vi "SVA 4MV6 T025(mimo) CCE.vi"() -> ()   [LabVIEW 2020]
uses:
  <vilib>/addons/Fuzzy Logic/TypeDefs/FL Defuzzification.ctl
  <vilib>/addons/Fuzzy Logic/TypeDefs/FL Antecedent Connective.ctl
  <vilib>/addons/Fuzzy Logic/TypeDefs/FL Consequent Implication.ctl
  <vilib>/addons/Fuzzy Logic/TypeDefs/FL Modifier.ctl
  <vilib>/addons/Fuzzy Logic/Membership/FL Create Membership Function (Triangle).vi
  <vilib>/addons/Fuzzy Logic/Membership/FL Create Membership Function (Trapezoid).vi
  <vilib>/addons/Fuzzy Logic/FL Fuzzy Controller (MIMO).vi
  <vilib>/addons/Fuzzy Logic/NI_Fuzzy_Logic_API.lvlib
panel:
  out "output values":dbl[](array[numeric])
  out "distancia":dbl(slide) scale=0.0..100.0
  out "angulo":dbl(knob) scale=-25.0..25.0
  in  "Reset":bool
  out "Motor Izquierda":dbl(slide) scale=-100.0..100.0
  out "Motor Derecha":dbl(slide) scale=-100.0..100.0
  out "Plano de trabajo":picture
  in  "stop":bool
  # "Ceballos Conde Emanuel\n4MV6\nSistemas de visión artificial\n2022/1"
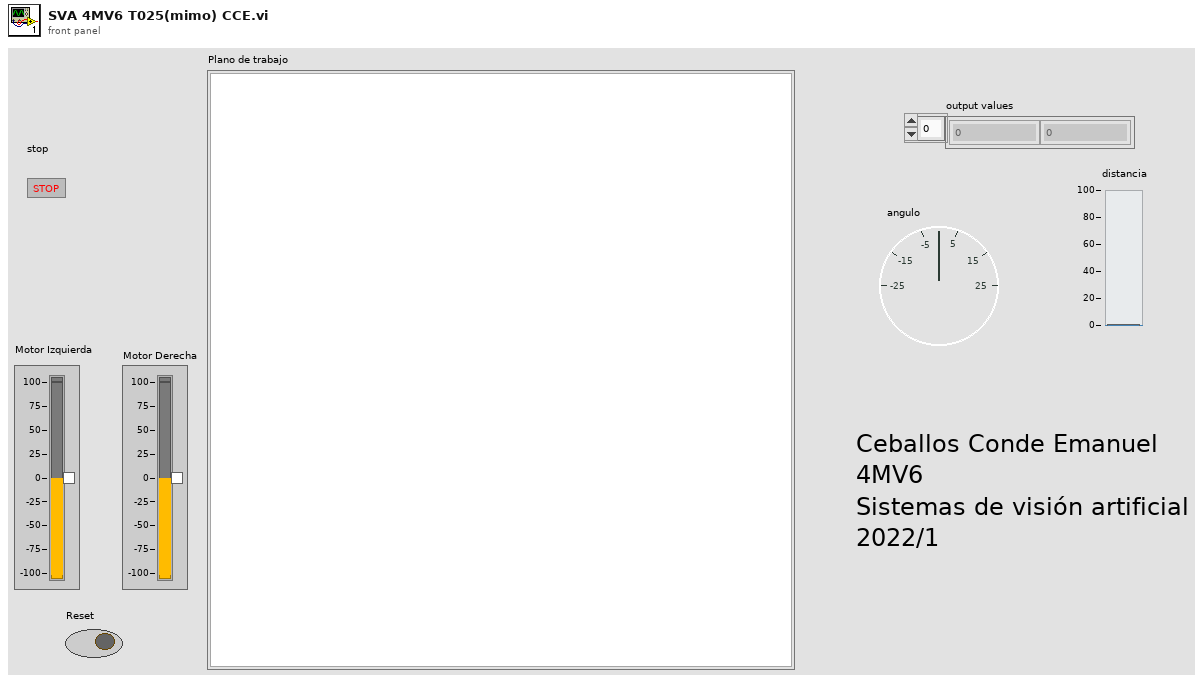
[diagram p1: front panel]
types:
  T1 = typedef "NI_Fuzzy_Logic_API.lvlib/FL Defuzzification.ctl" = u16
  T2 = typedef "NI_Fuzzy_Logic_API.lvlib/FL Membership Function.ctl" = cluster{"name":string, "shape":T3, "points":dbl[], "color":u32, "user-defined shape index":i32}
  T3 = typedef "NI_Fuzzy_Logic_API.lvlib/FL Membership Function Shape.ctl" = u16
  T4 = typedef "NI_Fuzzy_Logic_API.lvlib/FL Variable.ctl" = cluster{"name":string, "range":dbl[], "MFs":T2[]}
  T5 = typedef "NI_Fuzzy_Logic_API.lvlib/FL Modifier.ctl" = u16
  T6 = typedef "NI_Fuzzy_Logic_API.lvlib/FL Consequent Implication.ctl" = u16
  T7 = typedef "NI_Fuzzy_Logic_API.lvlib/FL Antecedent Connective.ctl" = u16
  T8 = typedef "NI_Fuzzy_Logic_API.lvlib/FL Consequent.ctl" = cluster{"Var Index":i32, "MF Index":i32, "Cond":T5}
  T9 = typedef "NI_Fuzzy_Logic_API.lvlib/FL Antecedent.ctl" = cluster{"Var Index":i32, "MF Index":i32, "Cond":T5}
  T10 = typedef "NI_Fuzzy_Logic_API.lvlib/FL Rule.ctl" = cluster{"antecedents":T9[], "antecedent connective":T7, "consequents":T8[], "consequent implication":T6, "degree of support":dbl}
  T11 = typedef "NI_Fuzzy_Logic_API.lvlib/FL System.ctl" = cluster{"input variables":T4[], "output variables":T4[], "rules":T10[], "defuzzification method":T1, "description":string, "user MF interpolating polynomials":T12[]}
  T12 = typedef "NI_Fuzzy_Logic_API.lvlib/FL Interpolating polynomials.ctl" = cluster{"X":dbl[], "Y":dbl[], "Y(x) coeff":dbl[][], "X(y) coeff":dbl[][], "Area(y) coeff":dbl[][], "coa_x(y) coeff":dbl[][]}
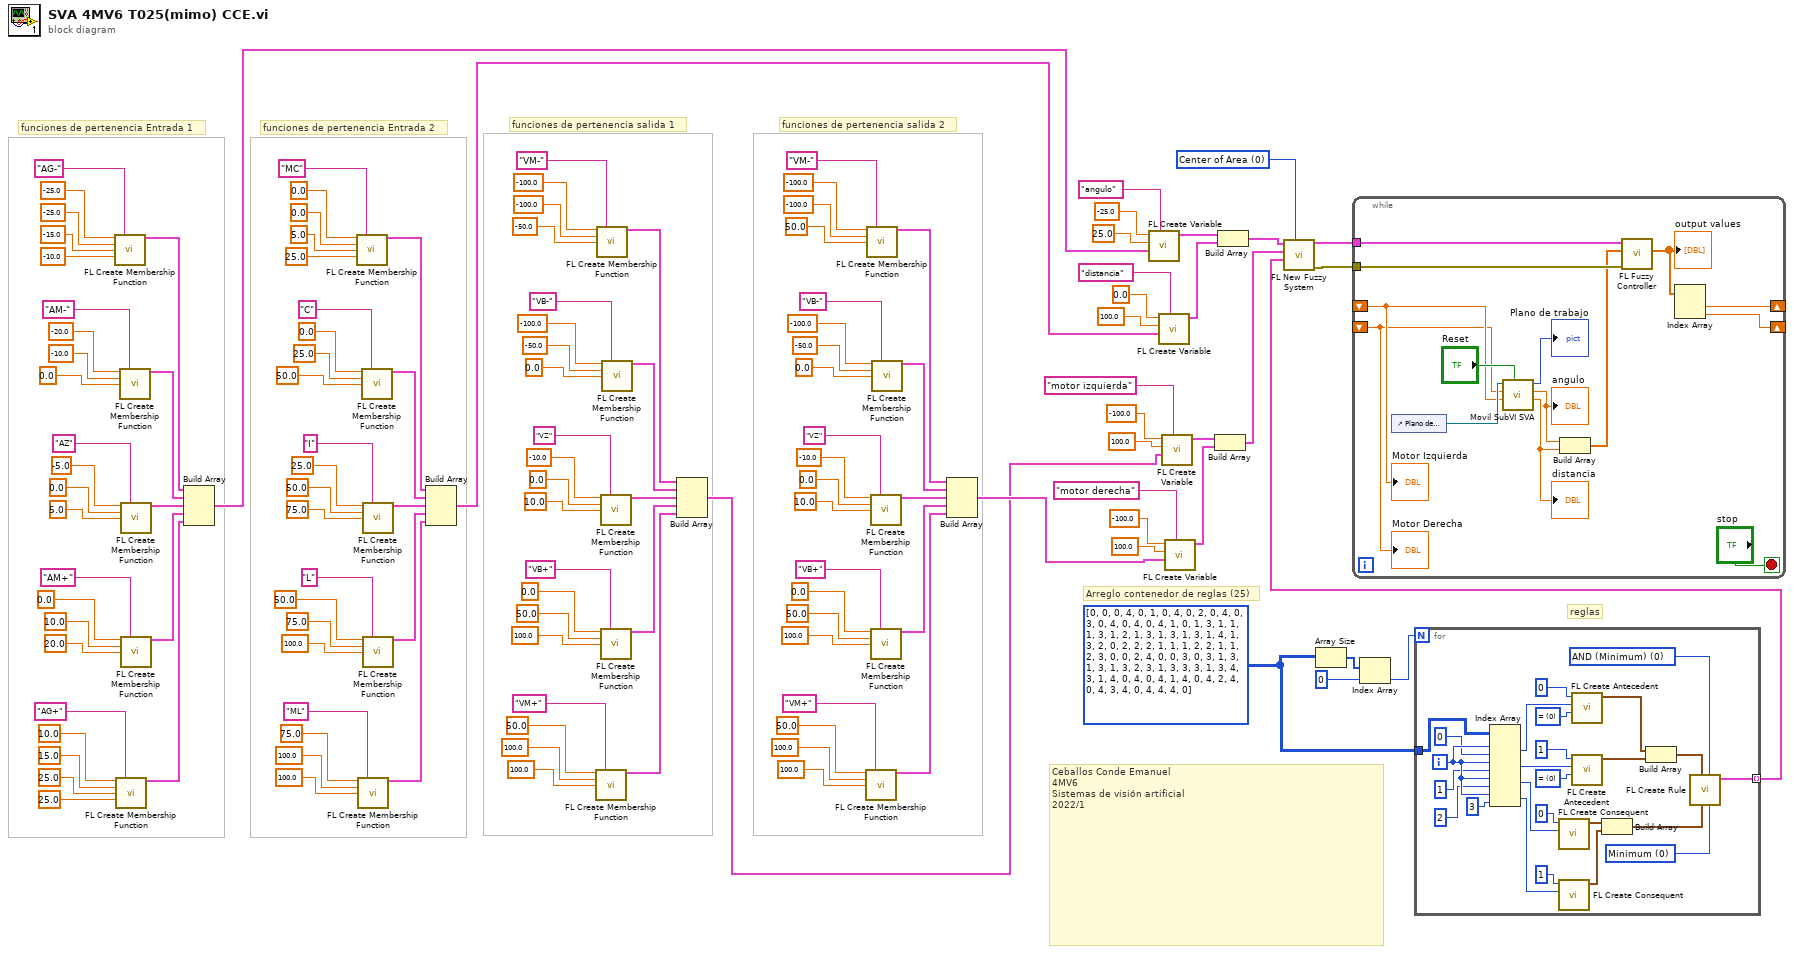
[diagram p0: block diagram]
diagram:
  w4 = i32[][] [[0, 0, 0, 4], [0, 1, 0, 4], [0, 2, 0, 4], [0, 3, 0, 4], [0, 4, 0, 4], [1, 0, 1, 3], [1, 1, 1, 3], [1, 2, 1, 3], [1, 3, 1, 3], [1, 4, 1, 3], [2, 0, 2, 2], [2, 1, 1, 1], [2, 2, 1, 1], [2, 3, 0, 0], [2, 4, 0, 0], [3, 0, 3, 1], [3, 1, 3, 1], [3, 2, 3, 1], [3, 3, 3, 1], [3, 4, 3, 1], [4, 0, 4, 0], [4, 1, 4, 0], [4, 2, 4, 0], [4, 3, 4, 0], [4, 4, 4, 0]]
  w131 = T1 0 items=["Center of Area", "Modified Center of Area", "Center of Sums", "Center of Maximum", "Mean of Maximum"] ("defuzzification method")
  # "Ceballos Conde Emanuel\n4MV6\nSistemas de visión artificial\n2022/1"
  # "Arreglo contenedor de reglas (25)"
  # "funciones de pertenencia salida 2"
  # "funciones de pertenencia salida 1"
  # "funciones de pertenencia Entrada 2"
  # "funciones de pertenencia Entrada 1"
  # "reglas"
  n1 = call-poly <vilib>:"FL Create Membership Function.vi"("left base"=-25.0, "name"="AG-", "left top"=-25.0 ("top"), "right top"=-15.0 ("right base"), "right base"=-10.0) -> ("membership function"=w107:T2)  [unwired: 9 in, 1 out]
  n2 = call-poly <vilib>:"FL Create Membership Function.vi"("left base"=10.0, "name"="AG+", "left top"=15.0 ("top"), "right top"=25.0 ("right base"), "right base"=25.0) -> ("membership function"=w87:T2)  [unwired: 9 in, 1 out]
  n3 = call-poly <vilib>:"FL Create Membership Function.vi"("left base"=-20.0, "name"="AM-", "top"=-10.0, "right base"=0.0) -> ("membership function"=w102:T2)  [unwired: 10 in, 1 out]
  n4 = call-poly <vilib>:"FL Create Membership Function.vi"("left base"=-5.0, "name"="AZ", "top"=0.0, "right base"=5.0) -> ("membership function"=w97:T2)  [unwired: 10 in, 1 out]
  n5 = call-poly <vilib>:"FL Create Membership Function.vi"("left base"=0.0, "name"="AM+", "top"=10.0, "right base"=20.0) -> ("membership function"=w92:T2)  [unwired: 10 in, 1 out]
  n6 = Build Array(w107, w102, w97, w92, w87) -> (w84:T2[])
  n7 = call-poly <vilib>:"FL Create Membership Function.vi"("left base"=0.0, "name"="MC", "left top"=0.0 ("top"), "right top"=5.0 ("right base"), "right base"=25.0) -> ("membership function"=w79:T2)  [unwired: 9 in, 1 out]
  n8 = call-poly <vilib>:"FL Create Membership Function.vi"("left base"=75.0, "name"="ML", "top"=100.0, "right base"=100.0) -> ("membership function"=w59:T2)  [unwired: 10 in, 1 out]
  n9 = call-poly <vilib>:"FL Create Membership Function.vi"("left base"=0.0, "name"="C", "top"=25.0, "right base"=50.0) -> ("membership function"=w74:T2)  [unwired: 10 in, 1 out]
  n10 = call-poly <vilib>:"FL Create Membership Function.vi"("left base"=25.0, "name"="I", "top"=50.0, "right base"=75.0) -> ("membership function"=w69:T2)  [unwired: 10 in, 1 out]
  n11 = call-poly <vilib>:"FL Create Membership Function.vi"("left base"=50.0, "name"="L", "top"=75.0, "right base"=100.0) -> ("membership function"=w64:T2)  [unwired: 10 in, 1 out]
  n12 = Build Array(w79, w74, w69, w64, w59) -> (w57:T2[])
  n13 = call-poly <vilib>:"FL Create Membership Function.vi"("left base"=50.0, "name"="VM+", "top"=100.0, "right base"=100.0) -> ("membership function"=w32:T2)  [unwired: 10 in, 1 out]
  n14 = call-poly <vilib>:"FL Create Membership Function.vi"("left base"=-100.0, "name"="VM-", "top"=-100.0, "right base"=-50.0) -> ("membership function"=w52:T2)  [unwired: 10 in, 1 out]
  n15 = call-poly <vilib>:"FL Create Membership Function.vi"("left base"=-10.0, "name"="VZ", "top"=0.0, "right base"=10.0) -> ("membership function"=w42:T2)  [unwired: 10 in, 1 out]
  n16 = call-poly <vilib>:"FL Create Membership Function.vi"("left base"=0.0, "name"="VB+", "top"=50.0, "right base"=100.0) -> ("membership function"=w37:T2)  [unwired: 10 in, 1 out]
  n17 = call-poly <vilib>:"FL Create Membership Function.vi"("left base"=-100.0, "name"="VB-", "top"=-50.0, "right base"=0.0) -> ("membership function"=w47:T2)  [unwired: 10 in, 1 out]
  n18 = Build Array(w52, w47, w42, w37, w32) -> (w5:T2[])
  n19 = call-poly <vilib>:"FL Create Membership Function.vi"("left base"=50.0, "name"="VM+", "top"=100.0, "right base"=100.0) -> ("membership function"=w7:T2)  [unwired: 10 in, 1 out]
  n20 = call-poly <vilib>:"FL Create Membership Function.vi"("left base"=-100.0, "name"="VM-", "top"=-100.0, "right base"=50.0) -> ("membership function"=w27:T2)  [unwired: 10 in, 1 out]
  n21 = call-poly <vilib>:"FL Create Membership Function.vi"("left base"=-10.0, "name"="VZ", "top"=0.0, "right base"=10.0) -> ("membership function"=w17:T2)  [unwired: 10 in, 1 out]
  n22 = call-poly <vilib>:"FL Create Membership Function.vi"("left base"=0.0, "name"="VB+", "top"=50.0, "right base"=100.0) -> ("membership function"=w12:T2)  [unwired: 10 in, 1 out]
  n23 = call-poly <vilib>:"FL Create Membership Function.vi"("left base"=-100.0, "name"="VB-", "top"=-50.0, "right base"=0.0) -> ("membership function"=w22:T2)  [unwired: 10 in, 1 out]
  n24 = Build Array(w27, w22, w17, w12, w7) -> (w6:T2[])
  n25 = call <vilib>:"FL Create Variable.vi"("name"="angulo", "membership functions"=w84, "maximum"=25.0, "minimum"=-25.0) -> ("variable"=w127:T4)  [unwired: 6 in, 1 out]
  n26 = call <vilib>:"FL Create Variable.vi"("name"="distancia", "membership functions"=w57, "maximum"=100.0, "minimum"=0.0) -> ("variable"=w114:T4)  [unwired: 6 in, 1 out]
  n27 = call <vilib>:"FL Create Variable.vi"("name"="motor izquierda", "membership functions"=w5, "maximum"=100.0, "minimum"=-100.0) -> ("variable"=w123:T4)  [unwired: 6 in, 1 out]
  n28 = call <vilib>:"FL Create Variable.vi"("name"="motor derecha", "membership functions"=w6, "maximum"=100.0, "minimum"=-100.0) -> ("variable"=w115:T4)  [unwired: 6 in, 1 out]
  n29 = Build Array(w123, w115) -> (w112:T4[])
  n30 = Build Array(w127, w114) -> (w113:T4[])
  n31 = Array Size(array=w4) -> (size(s)=w3:i32[])
  n32 = Index Array(array=w3, index=0) -> (element=w2:i32)
  n33 = for {
    N: w2 -> [_]
    tunnel: [w149] -> w119 mode=indexing
    tunnel: w4 -> [w134]
    i -> [w143]
    w147 = T5 0 items=["=", "!="] ("condition")
    w154 = T5 0 items=["=", "!="] ("condition")
    w157 = T6 0 items=["Minimum", "Product"] ("consequent implication")
    w158 = T7 0 items=["AND (Minimum)", "AND (Product)", "OR (Maximum)", "OR (Probabilistic)"] ("antecedent connective")
    n34 = Index Array(array=w134, index (row) #1=w143, index (col) #1=0 ("disabled index (col)"), index (row) #2=w143, index (col) #2=1 ("disabled index (col)"), index (row) #3=w143, index (col) #3=2 ("disabled index (col)"), index (row) #4=w143, index (col) #4=3 ("disabled index (col)")) -> (element #1=w138:i32, element #2=w137:i32, element #3=w136:i32, element #4=w135:i32)
    n35 = call <vilib>:"FL Create Consequent.vi"("membership function index"=w136, "variable index"=0) -> ("consequent"=w155:T8)  [unwired: 8 in, 1 out]
    n36 = call <vilib>:"FL Create Consequent.vi"("membership function index"=w135, "variable index"=1) -> ("consequent"=w144:T8)  [unwired: 8 in, 1 out]
    n37 = call <vilib>:"FL Create Antecedent.vi"("condition"=w154, "membership function index"=w138, "variable index"=0) -> ("antecedent"=w156:T9)  [unwired: 7 in, 1 out]
    n38 = call <vilib>:"FL Create Antecedent.vi"("condition"=w147, "membership function index"=w137, "variable index"=1) -> ("antecedent"=w146:T9)  [unwired: 7 in, 1 out]
    n39 = Build Array(w155, w144) -> (w150:T8[])
    n40 = Build Array(w156, w146) -> (w151:T9[])
    n41 = call <vilib>:"FL Create Rule.vi"("consequent implication"=w157, "antecedent connective"=w158, "consequents"=w150, "antecedents"=w151) -> ("rule"=w149:T10)  [unwired: 6 in, 1 out]
  }
  n42 = call <vilib>:"FL New Fuzzy System.vi"("defuzzification method"=w131, "rules"=w119, "output variables"=w112, "input variables"=w113) -> ("error out"=w132:errorcluster, "fuzzy system out"=w133:T11)  [unwired: 6 in]
  n43 = while {
    tunnel: w133 -> [w168]
    tunnel: w132 -> [w167]
    shift-right: [w165] -> _
    shift-left: _ -> [w163]
    shift-right: [w164] -> _
    shift-left: _ -> [w162]
    stop <- "stop" stop-if-true
    n44 = control-ref of="Plano de trabajo"() -> (w170:refnum<vi>)
    n45 = call "Movil SubVI SVA.vi"("Reset"="Reset", "Motor Izquierda"=w163, "Motor Derecha"=w162, "Ref Plano"=w170) -> ("Distancia"=w159:dbl, "Angulo"=w160:dbl, "Plano de trabajo"=→"Plano de trabajo":picture)  [unwired: 3 in, 2 out]
    "distancia" <- w159
    "angulo" <- w160
    n46 = Build Array(w160, w159) -> (w161:dbl[])
    n47 = call-poly <vilib>:"FL Fuzzy Controller.vi"("error in (no error)"=w167, "input values"=w161, "fuzzy system in"=w168) -> ("output values"=w166:dbl[])  [unwired: 4 in, 4 out]
    "output values" <- w166
    n48 = Index Array(array=w166) -> (element #1=w165:dbl, element #2=w164:dbl)  [unwired: 2 in]
    "Motor Derecha" <- w162
    "Motor Izquierda" <- w163
  }
